vi "QuP Multiplexer Control.vi"() -> ()   [LabVIEW 2020, in "QuPMXdriver.lvlib"]
uses:
  QuPMXdriver.lvlib
  91754cce-ab52-4237-b78a-64c01c446f44.vi
  32ad12f4-2c8c-4504-800a-0d774754ae80.vi
  bf4f7028-8ca7-4759-aadb-7144e2be3c91.vi
  040f1b57-66c1-4072-aa26-6ea72dd8171f.vi
  6aed5eb3-691d-4dc6-b830-00691c629857.vi
  3345cd23-f609-4396-914e-6427162a2d46.vi
  Sequence Editor.vi
  <vilib>/Comparison/Equal/Equal Functor/Equal Functor.lvclass
panel:
  in  "Init-reset":bool caption="Reset after connect:"
  in  "Init-idquery":bool=TRUE caption="ID query after connect:"
  out "FPdisAcon":refnum<vi>[](array[refnum])
  in  "Startup delay (ms)":u32=2000
  in  "disconnect":bool
  out "dummy for event \"check channels\"":bool
  in  "Set to sequence line:":i32=2 min=1 step=1
  in  "set sq line":bool
  out "Connected\nboards":bool[](array[boolean])
  in  "Get sq from MX":bool
  in  "Load sq to MX":bool
  in  "no sequences get":bool
  out "Number of sequence lines:":i32 min=0 step=1
  in  "sequence editor":bool
  out "Guards ref array":refnum<vi>[][](array[refnum])
  in  "G5C1":bool
  in  "G5C2":bool
  in  "G6C1":bool
  in  "G6C2":bool
  in  "G4C1":bool
  in  "G4C2":bool
  in  "G3C1":bool
  in  "G3C2":bool
  in  "G2C1":bool
  in  "G2C2":bool
  in  "G1C1":bool
  in  "G1C2":bool
  out "No. of connected slave boards:":u32
  out "Slaves ref array":refnum<vi>[][](array[refnum])
  in  "S5C1":bool
  in  "S5C2":bool
  in  "S6C1":bool
  in  "S6C2":bool
  in  "S4C1":bool
  in  "S4C2":bool
  in  "S3C1":bool
  in  "S3C2":bool
  in  "S2C1":bool
  in  "S2C2":bool
  in  "S1C1":bool
  in  "S1C2":bool
  in  "connect":bool
  in  "Get Status":bool
  out "Ready?":bool=TRUE
  out "Enabled":bool=TRUE
  in  "check channels":bool
  in  "delay get":bool
  in  "delay set":bool
  in  "Enable\nDelay (ms)":dbl=2.0 min=0.8
  in  "timer get":bool
  in  "timer set":bool
  in  "Timer (ms)":i32=1000 min=0 step=1
  in  "Trigger polarity":enum32{"Positive", "Negative"}(radio)
  in  "Trigger source":enum32{"Internal", "External"}(radio)
  out "FPenAcon":refnum<vi>[](array[refnum])
  in  "Operation":enum32{"Remote", "Local"}(radio)=enum."Local"
  out "ID:":string
  in  "reset":bool
  in  "clear":bool
  in  "stop":bool
  in  "start":bool
  in  "resume":bool
  in  "pause":bool
  in  "Close":bool
  out "error":errorcluster
  in  "VISA":refnum<visa-resource-name>
  # "Connect"
  # "Status"
  # "Channels"
  # "Properties"
  # "Slave boards"
  # "1       2      3      4      5      6"
  # "Channel 1"
  # "Channel 2"
  # "1       2      3      4      5      6"
  # "Guards"
  # "Channel 1"
  # "These are buttons,\nclick it!"
  # "Channel 2"
  # "Sequence"
  # "Error"
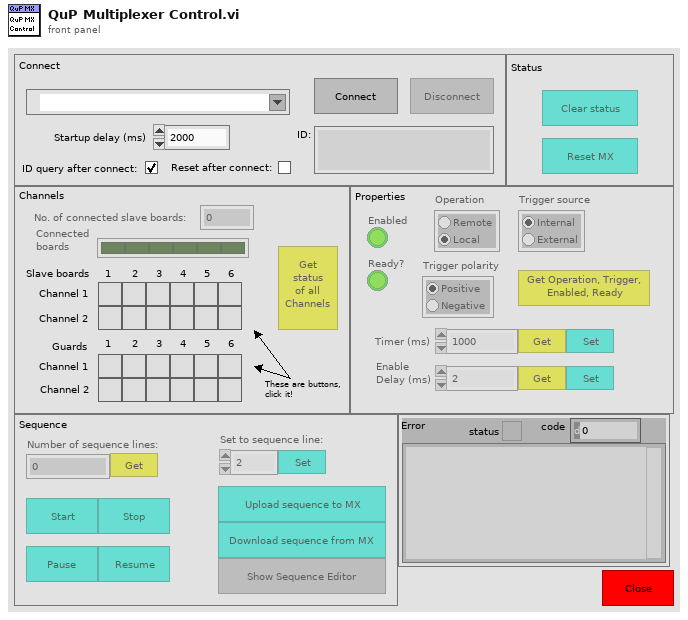
[diagram p1: front panel]
types:
  T1 = enum8{"Enabled", "Disabled", "Disabled and Grayed Out"}
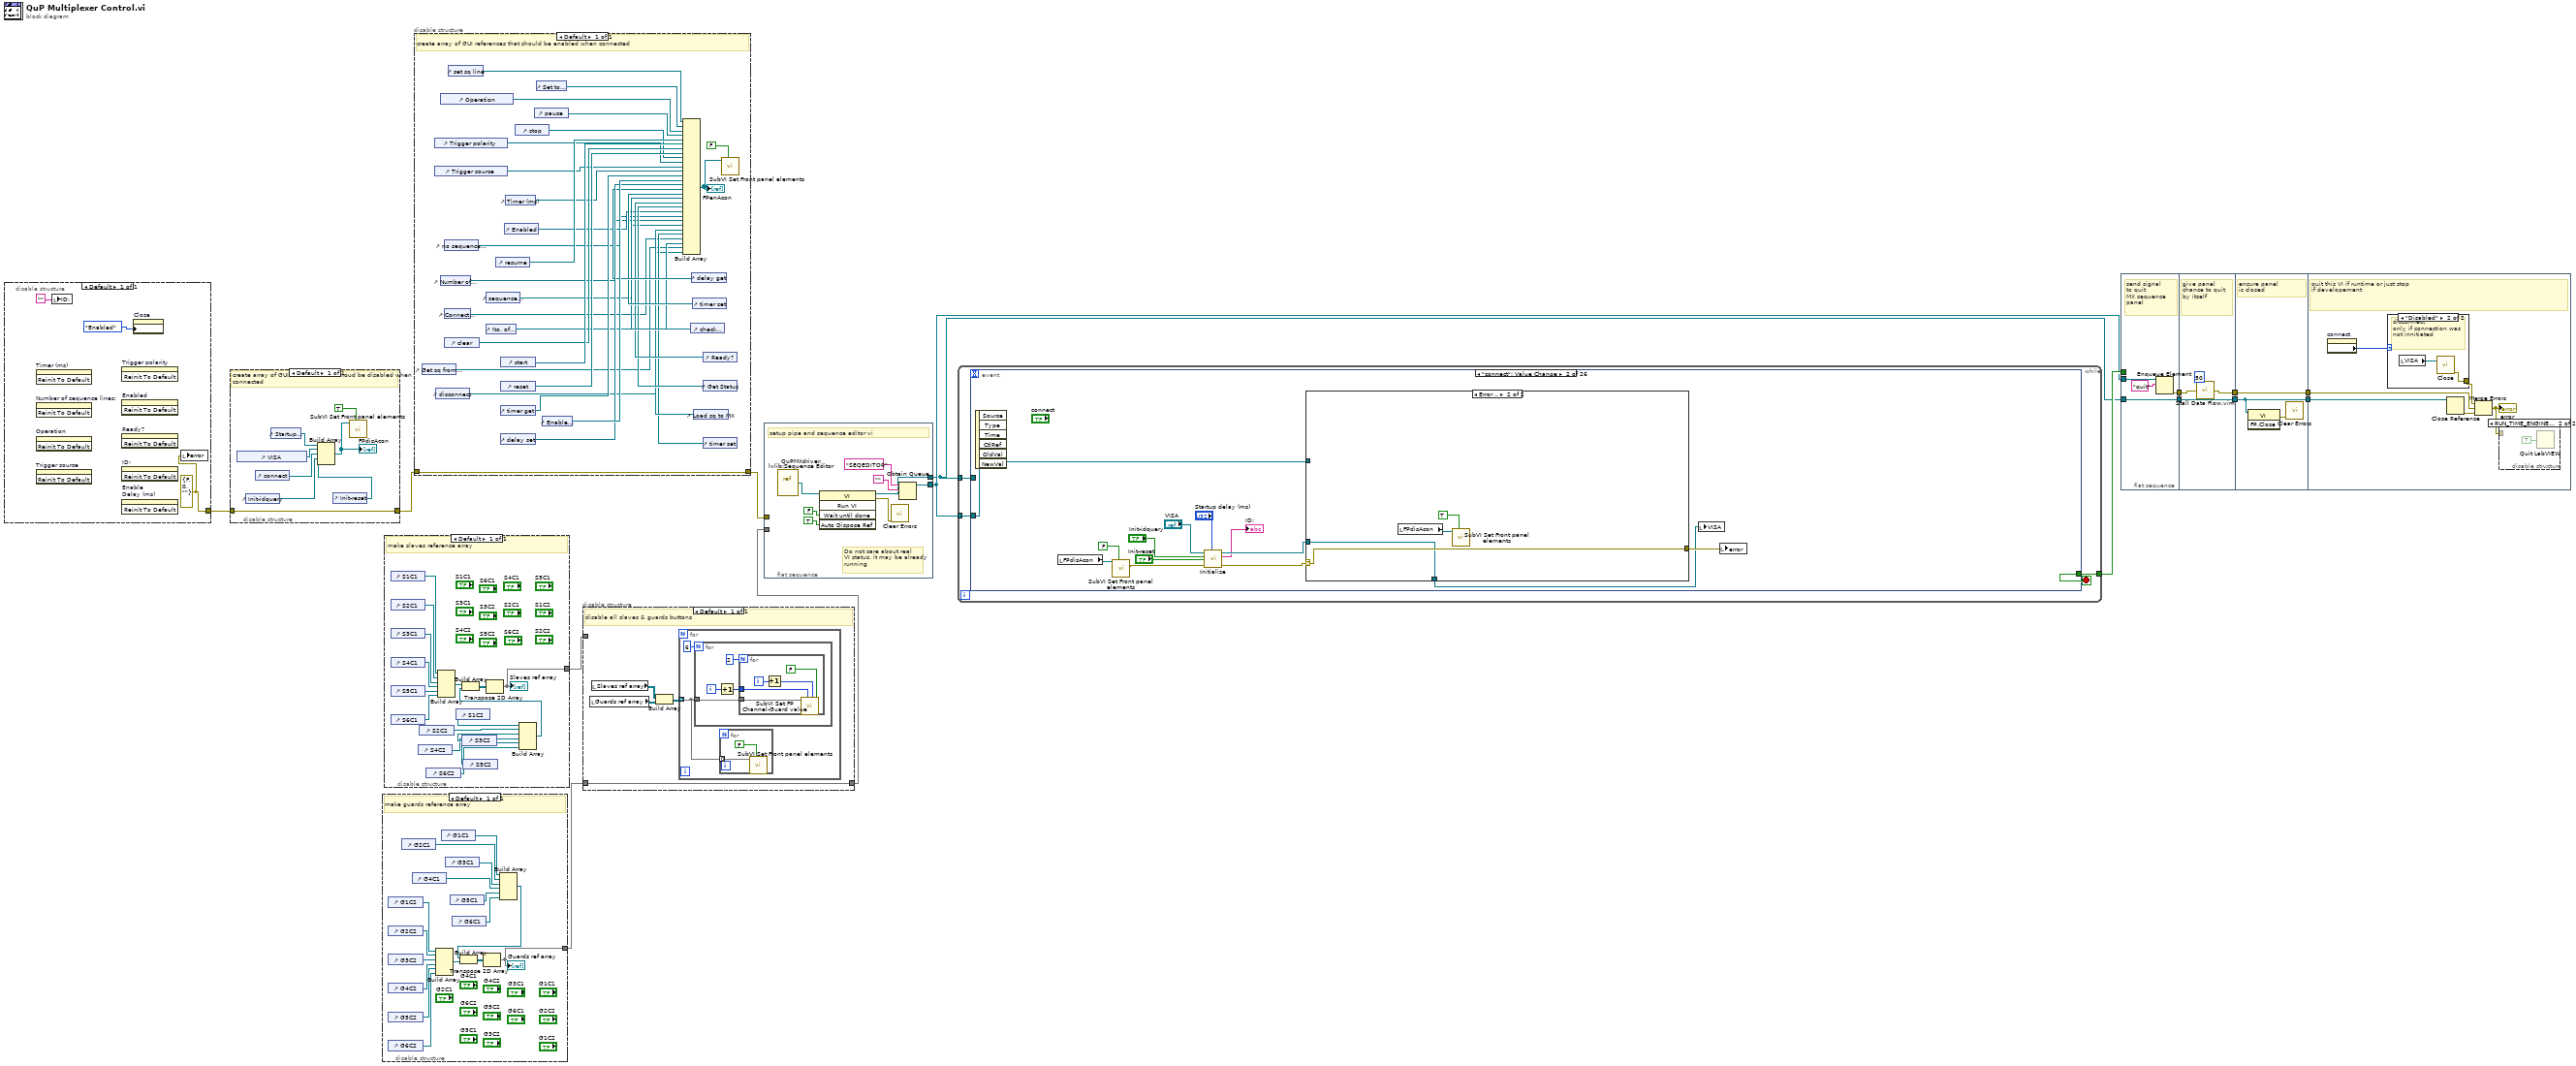
[diagram p0: block diagram]
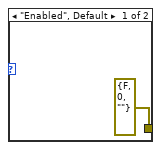
[diagram p2: hidden frame]
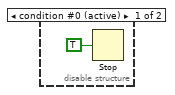
[diagram p3: hidden frame]
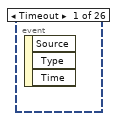
[diagram p4: hidden frame]
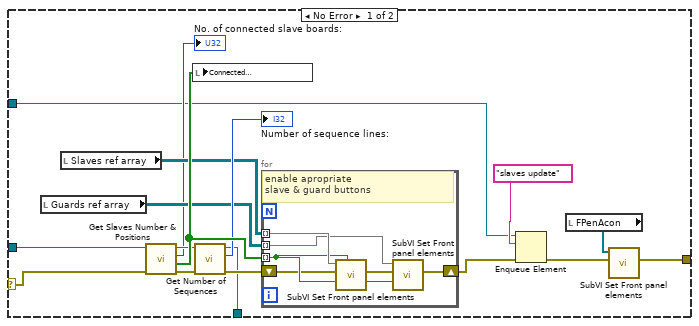
[diagram p5: hidden frame]
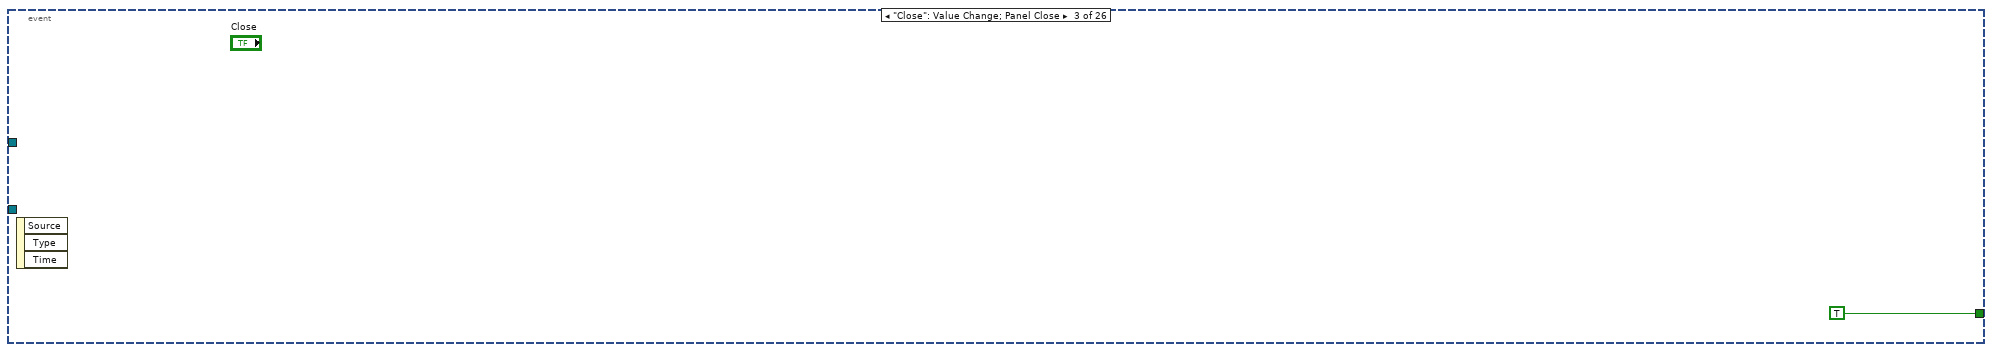
[diagram p6: hidden frame]
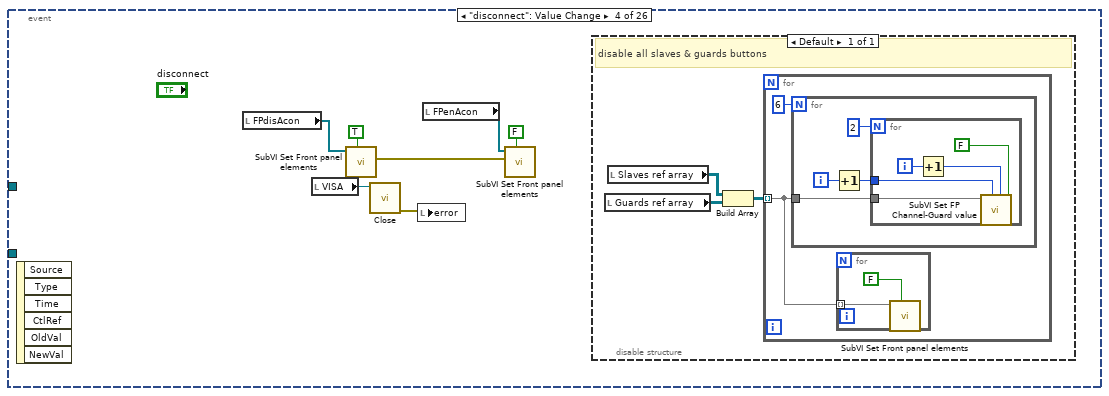
[diagram p7: hidden frame]
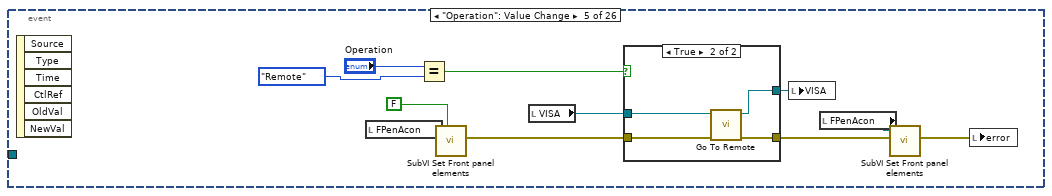
[diagram p8: hidden frame]
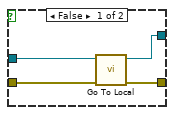
[diagram p9: hidden frame]
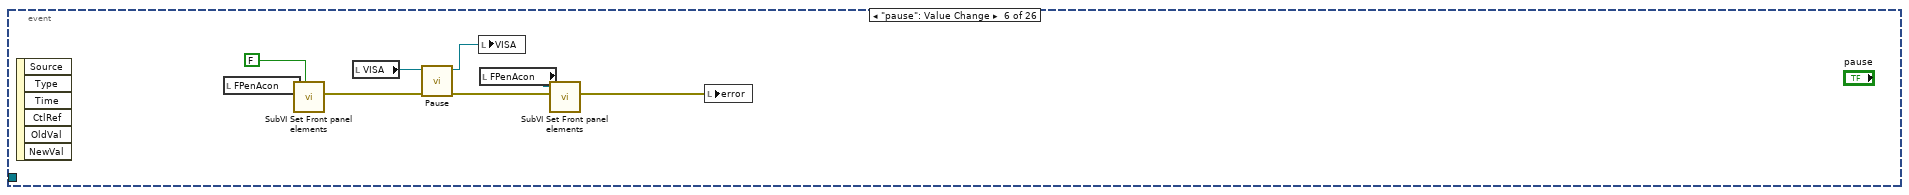
[diagram p10: hidden frame]
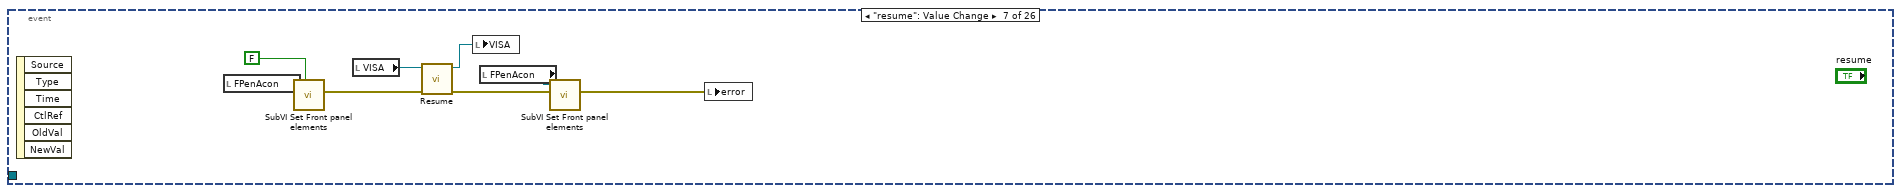
[diagram p11: hidden frame]
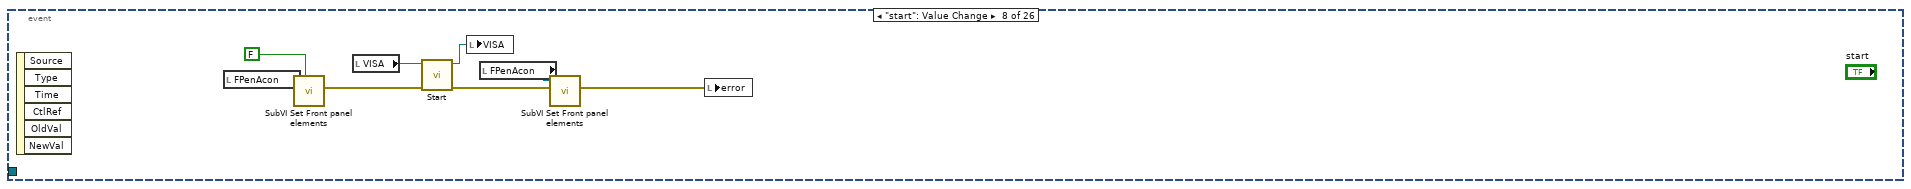
[diagram p12: hidden frame]
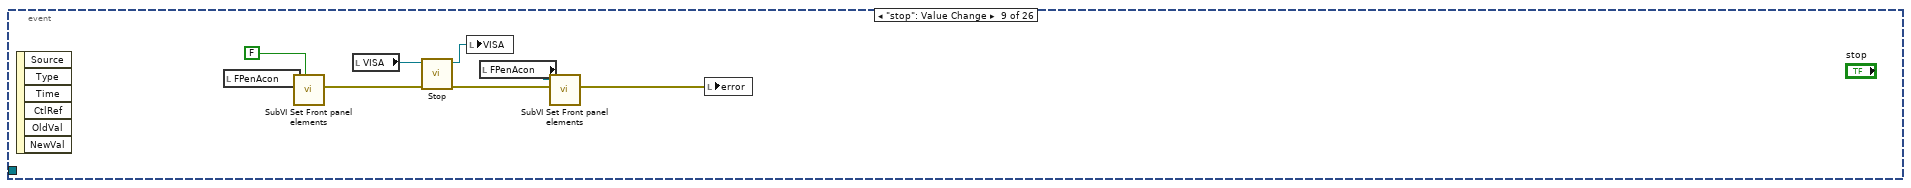
[diagram p13: hidden frame]
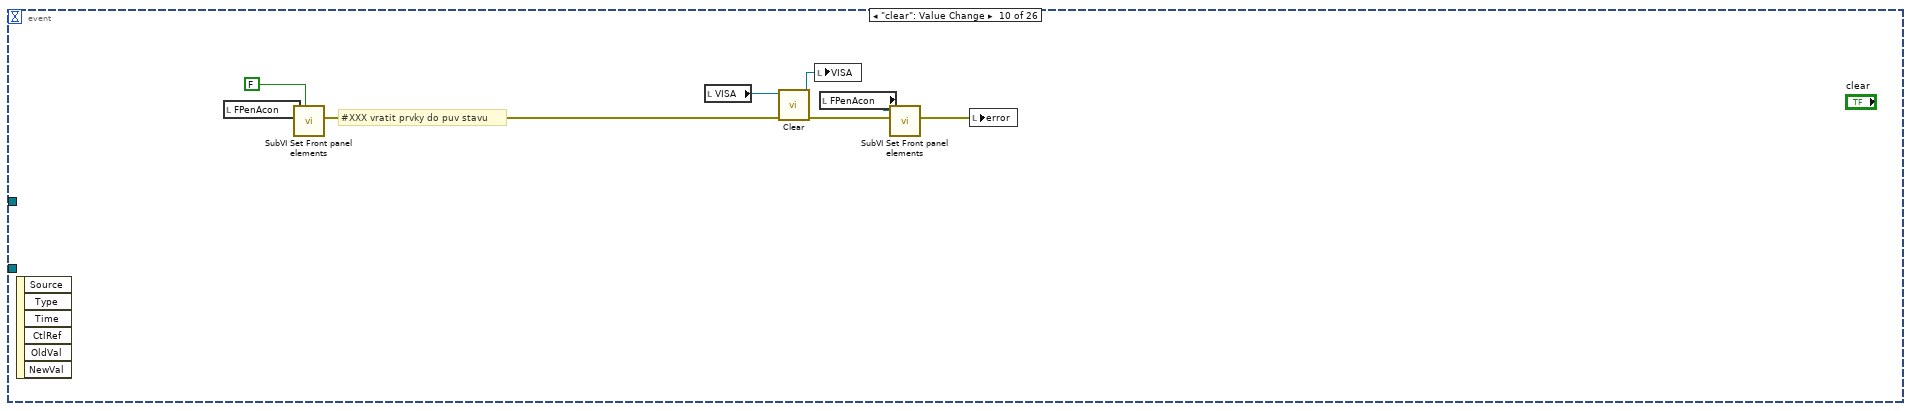
[diagram p14: hidden frame]
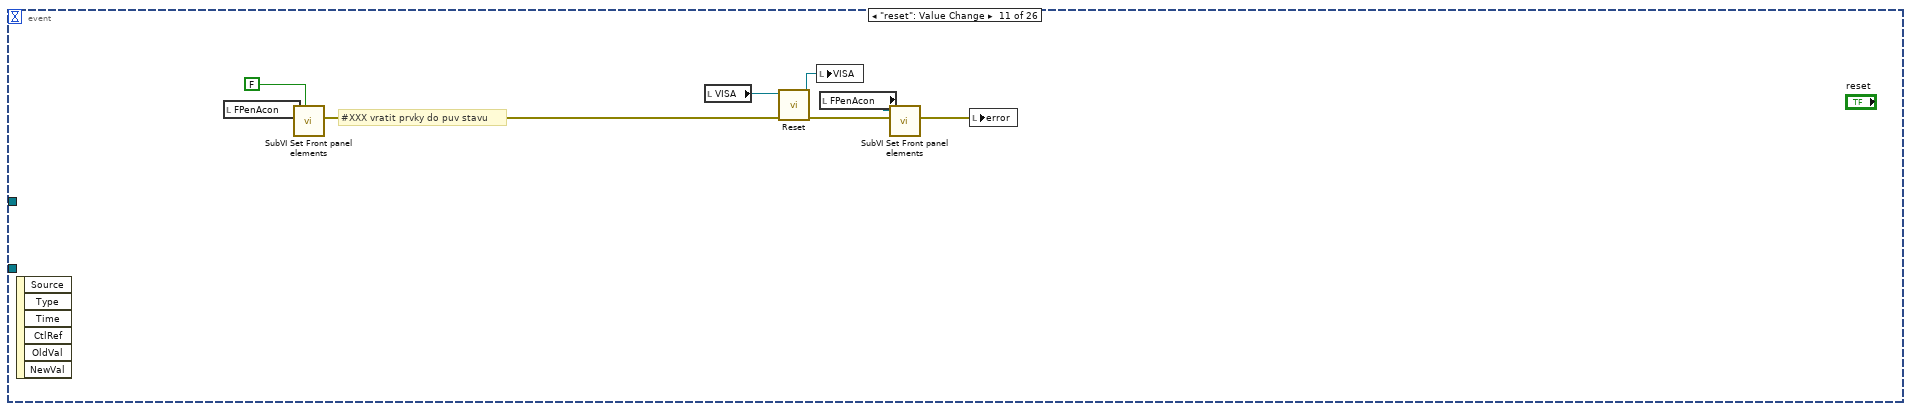
[diagram p15: hidden frame]
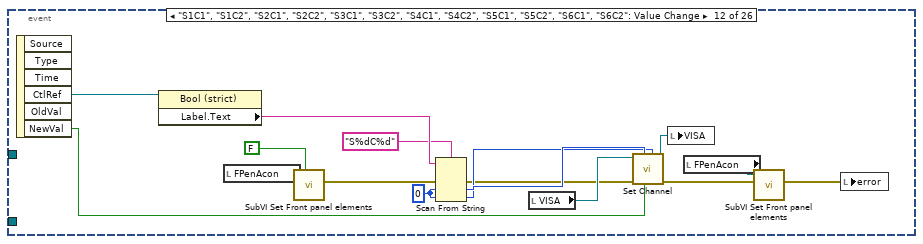
[diagram p16: hidden frame]
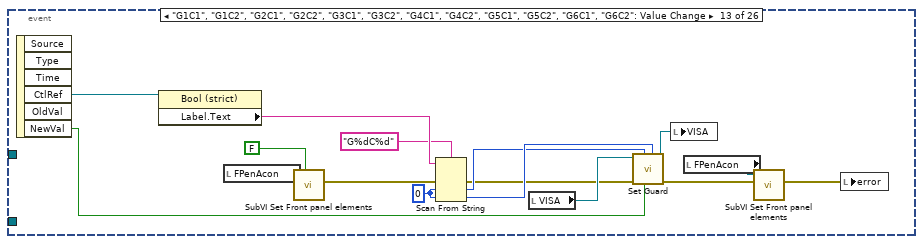
[diagram p17: hidden frame]
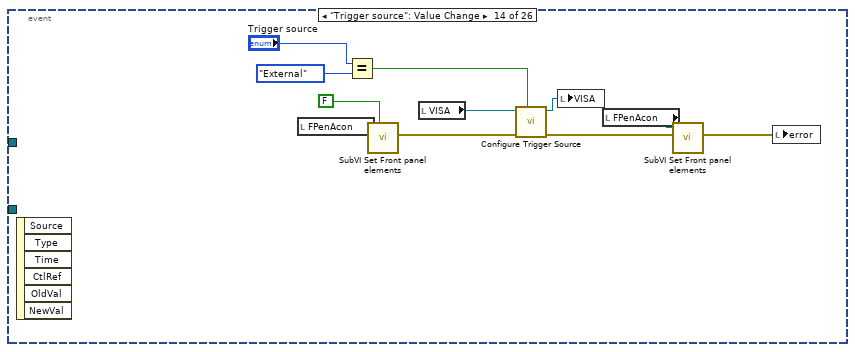
[diagram p18: hidden frame]
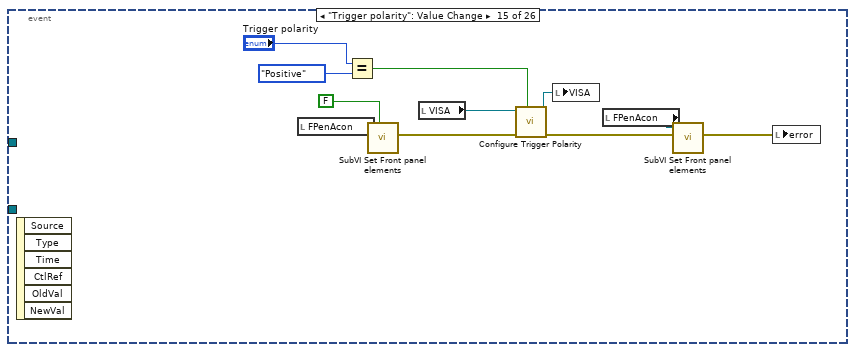
[diagram p19: hidden frame]
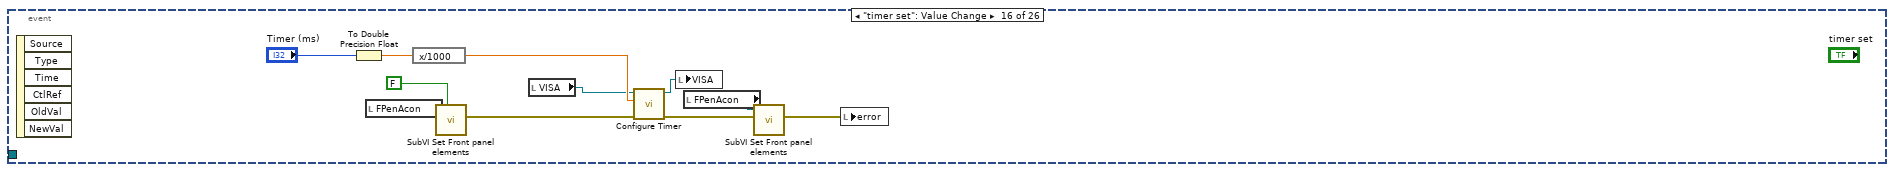
[diagram p20: hidden frame]
diagram:
  n1 = disable-structure shown="Default" {
    disable-tunnel: [w16] -> w5
    frame Enabled {
      w16 = errorcluster {"status"=FALSE, "code"=0, "source"=""} ("error in (no error)")
      n2 = invoke on="Timer (ms)" class="DigNum (strict)" method="Reinit To Default"() -> ()  [unwired: 3 in, 3 out]
      n3 = invoke on="Number of sequence lines:" class="DigNum (strict)" method="Reinit To Default"() -> ()  [unwired: 3 in, 3 out]
      n4 = invoke on="Operation" class="RadioBtnsControl (strict)" method="Reinit To Default"() -> ()  [unwired: 3 in, 3 out]
      n5 = invoke on="Trigger source" class="RadioBtnsControl (strict)" method="Reinit To Default"() -> ()  [unwired: 3 in, 3 out]
      n6 = local write "ID:"("") -> ()
      n7 = invoke on="Trigger polarity" class="RadioBtnsControl (strict)" method="Reinit To Default"() -> ()  [unwired: 3 in, 3 out]
      n8 = invoke on="Enabled" class="Bool (strict)" method="Reinit To Default"() -> ()  [unwired: 3 in, 3 out]
      n9 = invoke on="Ready?" class="Bool (strict)" method="Reinit To Default"() -> ()  [unwired: 3 in, 3 out]
      n10 = invoke on="ID:" class="Str" method="Reinit To Default"() -> ()  [unwired: 3 in, 3 out]
      n11 = invoke on="Enable\nDelay (ms)" class="DigNum (strict)" method="Reinit To Default"() -> ()  [unwired: 3 in, 3 out]
      n12 = property on="Close" class="Bool"("DisabledEnum"=T1."Enabled" ("Disabled")) -> ()  [unwired: 2 in, 2 out]
      n13 = local write "error"(w16) -> ()
    }
  }
  n14 = disable-structure shown="Default" {
    disable-tunnel: [w21] -> w6
    disable-tunnel: w5 -> [w21]
    frame Enabled {
      # "create array of GUI references that shoud be disabled when connected"
      n15 = control-ref of="VISA"() -> (w25:refnum<vi>)
      n16 = control-ref of="Init-idquery"() -> (w20:refnum<vi>)
      n17 = control-ref of="connect"() -> (w24:refnum<vi>)
      n18 = control-ref of="Startup delay (ms)"() -> (w26:refnum<vi>)
      n19 = control-ref of="Init-reset"() -> (w19:refnum<vi>)
      n20 = Build Array(w26, w25, w24, w20, w19) -> (w22:refnum<vi>[])
      "FPdisAcon" <- w22
      n21 = call "SubVI Set Front panel elements.vi"("Enable elements (T)"=TRUE ("Enable elements"), "Array"=w22) -> ()  [unwired: 9 in, 1 out]
    }
  }
  n22 = disable-structure shown="Default" {
    disable-tunnel: [w27] -> w13
    frame Enabled {
      # "make guards reference array"
      n23 = control-ref of="G1C2"() -> (w28:refnum<vi>)
      n24 = control-ref of="G2C2"() -> (w29:refnum<vi>)
      n25 = control-ref of="G3C2"() -> (w30:refnum<vi>)
      n26 = control-ref of="G4C2"() -> (w31:refnum<vi>)
      n27 = control-ref of="G5C2"() -> (w32:refnum<vi>)
      n28 = control-ref of="G6C2"() -> (w33:refnum<vi>)
      n29 = control-ref of="G2C1"() -> (w36:refnum<vi>)
      n30 = control-ref of="G4C1"() -> (w38:refnum<vi>)
      n31 = Build Array(w28, w29, w30, w31, w32, w33) -> (w41:refnum<vi>[])
      n32 = control-ref of="G1C1"() -> (w35:refnum<vi>)
      n33 = control-ref of="G3C1"() -> (w37:refnum<vi>)
      n34 = control-ref of="G5C1"() -> (w39:refnum<vi>)
      n35 = control-ref of="G6C1"() -> (w40:refnum<vi>)
      n36 = Build Array(w35, w36, w37, w38, w39, w40) -> (w34:refnum<vi>[])
      n37 = Build Array(w34, w41) -> (w42:refnum<vi>[][])
      n38 = Transpose 2D Array(2D array=w42) -> (transposed array=w27:refnum<vi>[][])
      "Guards ref array" <- w27
    }
  }
  n39 = disable-structure shown="Default" {
    disable-tunnel: [w43] -> w14
    frame Enabled {
      # "make slaves reference array"
      n40 = control-ref of="S1C1"() -> (w58:refnum<vi>)
      n41 = control-ref of="S2C1"() -> (w57:refnum<vi>)
      n42 = control-ref of="S3C1"() -> (w56:refnum<vi>)
      n43 = control-ref of="S4C1"() -> (w55:refnum<vi>)
      n44 = control-ref of="S5C1"() -> (w54:refnum<vi>)
      n45 = control-ref of="S6C1"() -> (w53:refnum<vi>)
      n46 = control-ref of="S4C2"() -> (w49:refnum<vi>)
      n47 = control-ref of="S2C2"() -> (w51:refnum<vi>)
      n48 = control-ref of="S6C2"() -> (w47:refnum<vi>)
      n49 = Build Array(w58, w57, w56, w55, w54, w53) -> (w45:refnum<vi>[])
      n50 = control-ref of="S1C2"() -> (w52:refnum<vi>)
      n51 = control-ref of="S3C2"() -> (w50:refnum<vi>)
      n52 = control-ref of="S5C2"() -> (w48:refnum<vi>)
      n53 = Build Array(w52, w51, w50, w49, w48, w47) -> (w46:refnum<vi>[])
      n54 = Build Array(w45, w46) -> (w44:refnum<vi>[][])
      n55 = Transpose 2D Array(2D array=w44) -> (transposed array=w43:refnum<vi>[][])
      "Slaves ref array" <- w43
    }
  }
  n56 = disable-structure shown="Default" {
    disable-tunnel: [w66] -> w9
    disable-tunnel: w6 -> [w66]
    frame Enabled {
      # "create array of GUI references that should be enabled when connected"
      n57 = control-ref of="Get sq from MX"() -> (w62:refnum<vi>)
      n58 = control-ref of="Trigger polarity"() -> (w82:refnum<vi>)
      n59 = control-ref of="Trigger source"() -> (w81:refnum<vi>)
      n60 = control-ref of="disconnect"() -> (w59:refnum<vi>)
      n61 = control-ref of="Operation"() -> (w91:refnum<vi>)
      n62 = control-ref of="Number of sequence lines:"() -> (w69:refnum<vi>)
      n63 = control-ref of="no sequences get"() -> (w70:refnum<vi>)
      n64 = control-ref of="Connected\nboards"() -> (w64:refnum<vi>)
      n65 = control-ref of="clear"() -> (w87:refnum<vi>)
      n66 = control-ref of="set sq line"() -> (w60:refnum<vi>)
      n67 = control-ref of="sequence editor"() -> (w68:refnum<vi>)
      n68 = control-ref of="No. of connected slave boards:"() -> (w63:refnum<vi>)
      n69 = control-ref of="resume"() -> (w89:refnum<vi>)
      n70 = control-ref of="start"() -> (w88:refnum<vi>)
      n71 = control-ref of="reset"() -> (w86:refnum<vi>)
      n72 = control-ref of="timer get"() -> (w79:refnum<vi>)
      n73 = control-ref of="delay set"() -> (w77:refnum<vi>)
      n74 = control-ref of="Enabled"() -> (w71:refnum<vi>)
      n75 = control-ref of="Timer (ms)"() -> (w80:refnum<vi>)
      n76 = control-ref of="stop"() -> (w83:refnum<vi>)
      n77 = control-ref of="pause"() -> (w90:refnum<vi>)
      n78 = control-ref of="Set to sequence line:"() -> (w61:refnum<vi>)
      n79 = control-ref of="Enable\nDelay (ms)"() -> (w78:refnum<vi>)
      n80 = control-ref of="check channels"() -> (w74:refnum<vi>)
      n81 = control-ref of="delay get"() -> (w76:refnum<vi>)
      n82 = control-ref of="timer set"() -> (w75:refnum<vi>)
      n83 = control-ref of="Load sq to MX"() -> (w67:refnum<vi>)
      n84 = control-ref of="Ready?"() -> (w73:refnum<vi>)
      n85 = control-ref of="Get Status"() -> (w72:refnum<vi>)
      n86 = control-ref of="timer set"() -> (w65:refnum<vi>)
      n87 = Build Array(w60, w61, w91, w90, w89, w88, w87, w86, w83, w82, w81, w80, w79, w78, w77, w76, w75, w74, w73, w72, w71, w70, w69, w68, w67, w65, w64, w63, w62, w59) -> (w85:refnum<vi>[])
      "FPenAcon" <- w85
      n88 = call "SubVI Set Front panel elements.vi"("Enable elements (T)"=FALSE ("Enable elements"), "Array"=w85) -> ()  [unwired: 9 in, 1 out]
    }
  }
  n89 = disable-structure shown="Default" {
    disable-tunnel: w14 -> [_]
    disable-tunnel: w13 -> [w92]
    disable-tunnel: [w92] -> w10
    frame Enabled {
      # "disable all slaves & guards buttons"
      n90 = local read "Guards ref array"() -> (w93:refnum<vi>[][])
      n91 = local read "Slaves ref array"() -> (w95:refnum<vi>[][])
      n92 = Build Array(w95, w93) -> (w94:refnum<vi>[][][])
      n93 = for {
        tunnel: w94 -> [w96] mode=indexing
        n94 = for {
          N: 6 -> [_]
          tunnel: w96 -> [w101]
          i -> [w99]
          n95 = Increment(x=w99) -> (x+1=w98:i32)
          n96 = for {
            N: 2 -> [_]
            tunnel: w101 -> [w106]
            tunnel: w98 -> [w104]
            i -> [w103]
            n97 = Increment(x=w103) -> (x+1=w102:i32)
            n98 = call "SubVI Set FP Channel-Guard value.vi"("Value"=FALSE, "Ch ID"=w102, "Slave ID"=w104, "Slaves ref array"=w106) -> ()  [unwired: 7 in, 1 out]
          }
        }
        n99 = for {
          tunnel: w96 -> [w108] mode=indexing
          n100 = call "SubVI Set Front panel elements.vi"("Enable elements (T)"=FALSE, "Array"=w108) -> ()  [unwired: 9 in, 1 out]
        }
      }
    }
  }
  n101 = flat-sequence {
    tunnel: [w110] -> w12
    tunnel: [w112] -> w11
    tunnel: w10 -> [_]
    tunnel: w9 -> [_]
    frame #0 {
      # "Do not care about real\nVI status, it may be already\nrunning"
      # "setup pipe and sequence editor vi"
      n102 = vi-ref "QuPMXdriver.lvlib:Sequence Editor.vi"() -> (w116:refnum<vi>)
      n103 = invoke class="VI" method="Run VI"(reference=w116, "Wait until done"=FALSE ("Wait Until Done"), "Auto Dispose Ref"=TRUE ("Wait Until Done")) -> (reference out=w112:refnum<vi>, error out=w109:errorcluster)  [unwired: 2 in, 3 out]
      n104 = call <vilib>:"Clear Errors.vi"("error in (no error)"=w109) -> ()  [unwired: 5 in, 2 out]
      n105 = Obtain Queue(name (unnamed)="SEQEDITOR", element data type="") -> (queue out=w110:refnum<queue>)  [unwired: 3 in, 2 out]
    }
  }
  n106 = while {
    tunnel: [w119] -> w15
    tunnel: w12 -> [w118]
    tunnel: w11 -> [w117]
    stop <- w119 stop-if-true
    n107 = event shown="[1] \"connect\": Value Change" {
      selector: _ -> [_ _ _ _ _ _ _ _ _ _ _ _ _ _ _ _ _ _ _ _ _ _ _ _ _ _]
      dyn-events: _ -> [_ _ _ _ _ _ _ _ _ _ _ _ _ _ _ _ _ _ _ _ _ _ _ _ _ _]
      timeout: _ -> [_ _ _ _ _ _ _ _ _ _ _ _ _ _ _ _ _ _ _ _ _ _ _ _ _ _]
      tunnel: [_ _ TRUE ("Stop") _ _ _ _ _ _ _ _ _ _ _ _ _ _ _ _ _ _ _ _ _ _ _] -> w119
      tunnel: w118 -> [_ w129 _ _ _ _ _ _ _ _ _ _ _ _ _ _ _ _ _ w350 _ _ w419 _ _ w499]
      tunnel: w117 -> [_ _ _ _ _ _ _ _ _ _ _ _ _ _ _ _ _ _ _ _ _ _ _ w424 w474 w502]
      event Timeout {
        n108 = event-data() -> ()  [unwired: 1 in, 3 out]
      }
      event "connect": Value Change {
        n109 = event-data() -> ()  [unwired: 1 in, 6 out]
        n110 = local read "FPdisAcon"() -> (w126:refnum<vi>[])
        n111 = call "SubVI Set Front panel elements.vi"("Enable elements (T)"=FALSE, "Array"=w126) -> ("error out"=w124:errorcluster)  [unwired: 9 in]
        n112 = call "Initialize.vi"("Startup delay (0 ms)"="Startup delay (ms)", "error in (no error)"=w124, "Reset (False)"="Init-reset", "ID Query (True)"="Init-idquery", "VISA resource name"="VISA") -> ("error out"=w123:errorcluster, "ID"=→"ID:":string, "VISA resource name out"=w131:refnum<visa-resource-name>)  [unwired: 4 in]
        n113 = case shown="Error .." w123 {
          selector: w123 -> [w134 w159]
          tunnel: w131 -> [w141 w156]
          tunnel: w129 -> [w136 _]
          tunnel: [w135 w159] -> w127
          tunnel: [w133 w156] -> w120
          frame No Error {
            n114 = local read "Guards ref array"() -> (w144:refnum<vi>[][])
            n115 = local read "Slaves ref array"() -> (w143:refnum<vi>[][])
            n116 = call "Get Slaves Number & Positions.vi"("error in (no error)"=w134, "VISA resource name"=w141) -> ("error out"=w145:errorcluster, "Connected Slaves"=w149:bool[], "No. of Slaves"=→"No. of connected slave boards:":u32, "VISA resource name out"=w147:refnum<visa-resource-name>)  [unwired: 6 in]
            n117 = local write "Connected\nboards"(w149) -> ()
            n118 = call "Get Number of Sequences.vi"("error in (no error)"=w145, "VISA resource name"=w147) -> ("error out"=w146:errorcluster, "Number of sequences"=→"Number of sequence lines:":i32, "VISA resource name out"=w133:refnum<visa-resource-name>)  [unwired: 7 in]
            n119 = for {
              tunnel: w143 -> [w155] mode=indexing
              tunnel: w149 -> [w153] mode=indexing
              tunnel: w144 -> [w154] mode=indexing
              shift-right: [w151] -> w137
              shift-left: w146 -> [w150]
              # "enable apropriate\nslave & guard buttons"
              n120 = call "SubVI Set Front panel elements.vi"("Enable elements (T)"=w153, "error in (passthrough)"=w150, "Array"=w155) -> ("error out"=w152:errorcluster)  [unwired: 8 in]
              n121 = call "SubVI Set Front panel elements.vi"("Enable elements (T)"=w153, "error in (passthrough)"=w152, "Array"=w154) -> ("error out"=w151:errorcluster)  [unwired: 8 in]
            }
            n122 = Enqueue Element(queue=w136, element="slaves update", error in (no error)=w137) -> (error out=w140:errorcluster)  [unwired: 1 in, 2 out]
            n123 = local read "FPenAcon"() -> (w139:refnum<vi>[])
            n124 = call "SubVI Set Front panel elements.vi"("error in (passthrough)"=w140, "Array"=w139) -> ("error out"=w135:errorcluster)  [unwired: 9 in]
          }
          frame Error {
            n125 = local read "FPdisAcon"() -> (w157:refnum<vi>[])
            n126 = call "SubVI Set Front panel elements.vi"("Enable elements (T)"=TRUE, "Array"=w157) -> ()  [unwired: 9 in, 1 out]
          }
        }
        n127 = local write "VISA"(w120) -> ()
        n128 = local write "error"(w127) -> ()
      }
      event "Close": Value Change; Panel Close {
        n129 = event-data() -> ()  [unwired: 1 in, 3 out]
      }
      event "disconnect": Value Change {
        n130 = event-data() -> ()  [unwired: 1 in, 6 out]
        n131 = local read "FPdisAcon"() -> (w162:refnum<vi>[])
        n132 = local read "VISA"() -> (w167:refnum<visa-resource-name>)
        n133 = call "SubVI Set Front panel elements.vi"("Enable elements (T)"=TRUE, "Array"=w162) -> ("error out"=w163:errorcluster)  [unwired: 9 in]
        n134 = call "Close.vi"("VISA resource name"=w167) -> ("error out"=w166:errorcluster)  [unwired: 10 in]
        n135 = local write "error"(w166) -> ()
        n136 = local read "FPenAcon"() -> (w165:refnum<vi>[])
        n137 = call "SubVI Set Front panel elements.vi"("Enable elements (T)"=FALSE, "error in (passthrough)"=w163, "Array"=w165) -> ()  [unwired: 8 in, 1 out]
        n138 = disable-structure shown="Default" {
          frame Enabled {
            # "disable all slaves & guards buttons"
            n139 = local read "Guards ref array"() -> (w168:refnum<vi>[][])
            n140 = local read "Slaves ref array"() -> (w170:refnum<vi>[][])
            n141 = Build Array(w170, w168) -> (w169:refnum<vi>[][][])
            n142 = for {
              tunnel: w169 -> [w171] mode=indexing
              n143 = for {
                N: 6 -> [_]
                tunnel: w171 -> [w176]
                i -> [w174]
                n144 = Increment(x=w174) -> (x+1=w173:i32)
                n145 = for {
                  N: 2 -> [_]
                  tunnel: w176 -> [w181]
                  tunnel: w173 -> [w179]
                  i -> [w178]
                  n146 = Increment(x=w178) -> (x+1=w177:i32)
                  n147 = call "SubVI Set FP Channel-Guard value.vi"("Value"=FALSE, "Ch ID"=w177, "Slave ID"=w179, "Slaves ref array"=w181) -> ()  [unwired: 7 in, 1 out]
                }
              }
              n148 = for {
                tunnel: w171 -> [w183] mode=indexing
                n149 = call "SubVI Set Front panel elements.vi"("Enable elements (T)"=FALSE, "Array"=w183) -> ()  [unwired: 9 in, 1 out]
              }
            }
          }
        }
      }
      event "Operation": Value Change {
        n150 = event-data() -> ()  [unwired: 1 in, 6 out]
        n151 = local read "FPenAcon"() -> (w190:refnum<vi>[])
        n152 = Equal?(x="Operation", y=enum32{"Remote", "Local"}."Remote") -> (x = y?=w191:bool)
        n153 = call "SubVI Set Front panel elements.vi"("Enable elements (T)"=FALSE, "Array"=w190) -> ("error out"=w188:errorcluster)  [unwired: 9 in]
        n154 = local read "VISA"() -> (w194:refnum<visa-resource-name>)
        n155 = case shown="True" w191 {
          tunnel: [w198 w202] -> w187
          tunnel: w194 -> [w197 w201]
          tunnel: w188 -> [w196 w200]
          tunnel: [w195 w199] -> w184
          frame False {
            n156 = call "Go To Local.vi"("error in (no error)"=w196, "VISA resource name"=w197) -> ("error out"=w198:errorcluster, "VISA resource name out"=w195:refnum<visa-resource-name>)  [unwired: 8 in]
          }
          frame True {
            n157 = call "Go To Remote.vi"("error in (no error)"=w200, "VISA resource name"=w201) -> ("error out"=w202:errorcluster, "VISA resource name out"=w199:refnum<visa-resource-name>)  [unwired: 8 in]
          }
        }
        n158 = local write "VISA"(w184) -> ()
        n159 = local read "FPenAcon"() -> (w185:refnum<vi>[])
        n160 = call "SubVI Set Front panel elements.vi"("error in (passthrough)"=w187, "Array"=w185) -> ("error out"=w186:errorcluster)  [unwired: 9 in]
        n161 = local write "error"(w186) -> ()
      }
      event "pause": Value Change {
        n162 = event-data() -> ()  [unwired: 1 in, 6 out]
        n163 = local read "FPenAcon"() -> (w209:refnum<vi>[])
        n164 = call "SubVI Set Front panel elements.vi"("Enable elements (T)"=FALSE, "Array"=w209) -> ("error out"=w206:errorcluster)  [unwired: 9 in]
        n165 = local read "VISA"() -> (w210:refnum<visa-resource-name>)
        n166 = call "Pause.vi"("error in (no error)"=w206, "VISA resource name"=w210) -> ("error out"=w205:errorcluster, "VISA resource name out"=w203:refnum<visa-resource-name>)  [unwired: 8 in]
        n167 = local write "VISA"(w203) -> ()
        n168 = local read "FPenAcon"() -> (w207:refnum<vi>[])
        n169 = call "SubVI Set Front panel elements.vi"("error in (passthrough)"=w205, "Array"=w207) -> ("error out"=w204:errorcluster)  [unwired: 9 in]
        n170 = local write "error"(w204) -> ()
      }
      event "resume": Value Change {
        n171 = event-data() -> ()  [unwired: 1 in, 6 out]
        n172 = local read "FPenAcon"() -> (w216:refnum<vi>[])
        n173 = call "SubVI Set Front panel elements.vi"("Enable elements (T)"=FALSE, "Array"=w216) -> ("error out"=w214:errorcluster)  [unwired: 9 in]
        n174 = local read "VISA"() -> (w218:refnum<visa-resource-name>)
        n175 = call "Resume.vi"("error in (no error)"=w214, "VISA resource name"=w218) -> ("error out"=w213:errorcluster, "VISA resource name out"=w211:refnum<visa-resource-name>)  [unwired: 8 in]
        n176 = local write "VISA"(w211) -> ()
        n177 = local read "FPenAcon"() -> (w217:refnum<vi>[])
        n178 = call "SubVI Set Front panel elements.vi"("error in (passthrough)"=w213, "Array"=w217) -> ("error out"=w212:errorcluster)  [unwired: 9 in]
        n179 = local write "error"(w212) -> ()
      }
      event "start": Value Change {
        n180 = event-data() -> ()  [unwired: 1 in, 6 out]
        n181 = local read "FPenAcon"() -> (w224:refnum<vi>[])
        n182 = call "SubVI Set Front panel elements.vi"("Enable elements (T)"=FALSE, "Array"=w224) -> ("error out"=w222:errorcluster)  [unwired: 9 in]
        n183 = local read "VISA"() -> (w226:refnum<visa-resource-name>)
        n184 = call "Start.vi"("error in (no error)"=w222, "VISA resource name"=w226) -> ("error out"=w221:errorcluster, "VISA resource name out"=w219:refnum<visa-resource-name>)  [unwired: 8 in]
        n185 = local write "VISA"(w219) -> ()
        n186 = local read "FPenAcon"() -> (w225:refnum<vi>[])
        n187 = call "SubVI Set Front panel elements.vi"("error in (passthrough)"=w221, "Array"=w225) -> ("error out"=w220:errorcluster)  [unwired: 9 in]
        n188 = local write "error"(w220) -> ()
      }
      event "stop": Value Change {
        n189 = event-data() -> ()  [unwired: 1 in, 6 out]
        n190 = local read "FPenAcon"() -> (w232:refnum<vi>[])
        n191 = call "SubVI Set Front panel elements.vi"("Enable elements (T)"=FALSE, "Array"=w232) -> ("error out"=w230:errorcluster)  [unwired: 9 in]
        n192 = local read "VISA"() -> (w234:refnum<visa-resource-name>)
        n193 = call "Stop.vi"("error in (no error)"=w230, "VISA resource name"=w234) -> ("error out"=w229:errorcluster, "VISA resource name out"=w227:refnum<visa-resource-name>)  [unwired: 8 in]
        n194 = local write "VISA"(w227) -> ()
        n195 = local read "FPenAcon"() -> (w233:refnum<vi>[])
        n196 = call "SubVI Set Front panel elements.vi"("error in (passthrough)"=w229, "Array"=w233) -> ("error out"=w228:errorcluster)  [unwired: 9 in]
        n197 = local write "error"(w228) -> ()
      }
      event "clear": Value Change {
        # "#XXX vratit prvky do puv stavu"
        n198 = event-data() -> ()  [unwired: 1 in, 6 out]
        n199 = local read "FPenAcon"() -> (w240:refnum<vi>[])
        n200 = call "SubVI Set Front panel elements.vi"("Enable elements (T)"=FALSE, "Array"=w240) -> ("error out"=w238:errorcluster)  [unwired: 9 in]
        n201 = local read "VISA"() -> (w242:refnum<visa-resource-name>)
        n202 = call "Clear.vi"("error in (no error)"=w238, "VISA resource name"=w242) -> ("error out"=w237:errorcluster, "VISA resource name out"=w235:refnum<visa-resource-name>)  [unwired: 8 in]
        n203 = local write "VISA"(w235) -> ()
        n204 = local read "FPenAcon"() -> (w241:refnum<vi>[])
        n205 = call "SubVI Set Front panel elements.vi"("error in (passthrough)"=w237, "Array"=w241) -> ("error out"=w236:errorcluster)  [unwired: 9 in]
        n206 = local write "error"(w236) -> ()
      }
      event "reset": Value Change {
        # "#XXX vratit prvky do puv stavu"
        n207 = event-data() -> ()  [unwired: 1 in, 6 out]
        n208 = local read "FPenAcon"() -> (w248:refnum<vi>[])
        n209 = call "SubVI Set Front panel elements.vi"("Enable elements (T)"=FALSE, "Array"=w248) -> ("error out"=w246:errorcluster)  [unwired: 9 in]
        n210 = local read "VISA"() -> (w250:refnum<visa-resource-name>)
        n211 = call "Reset.vi"("error in (no error)"=w246, "VISA resource name"=w250) -> ("error out"=w245:errorcluster, "VISA resource name out"=w243:refnum<visa-resource-name>)  [unwired: 8 in]
        n212 = local write "VISA"(w243) -> ()
        n213 = local read "FPenAcon"() -> (w249:refnum<vi>[])
        n214 = call "SubVI Set Front panel elements.vi"("error in (passthrough)"=w245, "Array"=w249) -> ("error out"=w244:errorcluster)  [unwired: 9 in]
        n215 = local write "error"(w244) -> ()
      }
      event "S1C1", "S1C2", "S2C1", "S2C2", "S3C1", "S3C2", "S4C1", "S4C2", "S5C1", "S5C2", "S6C1", "S6C2": Value Change {
        w252 = 0 ("default value 1")
        n216 = event-data() -> ("CtlRef"=w266:refnum<vi>, "NewVal"=w260:bool)  [unwired: 1 in, 4 out]
        n217 = property class="Bool (strict)"(reference=w266) -> ("Label.Text"=w265:string)  [unwired: 1 in, 2 out]
        n218 = local read "FPenAcon"() -> (w255:refnum<vi>[])
        n219 = call "SubVI Set Front panel elements.vi"("Enable elements (T)"=FALSE, "Array"=w255) -> ("error out"=w253:errorcluster)  [unwired: 9 in]
        n220 = Scan From String(format string="S%dC%d", input string=w265, error in=w253, default 1=w252, default 2=w252) -> (error out=w259:errorcluster, output 1=w263:i32, output 2=w262:i32)  [unwired: 1 in, 2 out]
        n221 = local read "VISA"() -> (w261:refnum<visa-resource-name>)
        n222 = call "Set Channel.vi"("Channel"=w262, "Channel Status"=w260, "Slave"=w263, "error in (no error)"=w259, "VISA resource name"=w261) -> ("error out"=w257:errorcluster, "VISA resource name out"=w251:refnum<visa-resource-name>)  [unwired: 5 in]
        n223 = local write "VISA"(w251) -> ()
        n224 = local read "FPenAcon"() -> (w258:refnum<vi>[])
        n225 = call "SubVI Set Front panel elements.vi"("error in (passthrough)"=w257, "Array"=w258) -> ("error out"=w256:errorcluster)  [unwired: 9 in]
        n226 = local write "error"(w256) -> ()
      }
      event "G1C1", "G1C2", "G2C1", "G2C2", "G3C1", "G3C2", "G4C1", "G4C2", "G5C1", "G5C2", "G6C1", "G6C2": Value Change {
        w274 = 0 ("default value 1")
        n227 = event-data() -> ("CtlRef"=w280:refnum<vi>, "NewVal"=w276:bool)  [unwired: 1 in, 4 out]
        n228 = property class="Bool (strict)"(reference=w280) -> ("Label.Text"=w282:string)  [unwired: 1 in, 2 out]
        n229 = local read "FPenAcon"() -> (w273:refnum<vi>[])
        n230 = call "SubVI Set Front panel elements.vi"("Enable elements (T)"=FALSE, "Array"=w273) -> ("error out"=w271:errorcluster)  [unwired: 9 in]
        n231 = Scan From String(format string="G%dC%d", input string=w282, error in=w271, default 1=w274, default 2=w274) -> (error out=w275:errorcluster, output 1=w278:i32, output 2=w279:i32)  [unwired: 1 in, 2 out]
        n232 = local read "VISA"() -> (w277:refnum<visa-resource-name>)
        n233 = call "Set Guard.vi"("Channel"=w279, "Channel Guard Status"=w276, "Slave"=w278, "error in (no error)"=w275, "VISA resource name"=w277) -> ("error out"=w269:errorcluster, "VISA resource name out"=w267:refnum<visa-resource-name>)  [unwired: 5 in]
        n234 = local write "VISA"(w267) -> ()
        n235 = local read "FPenAcon"() -> (w270:refnum<vi>[])
        n236 = call "SubVI Set Front panel elements.vi"("error in (passthrough)"=w269, "Array"=w270) -> ("error out"=w268:errorcluster)  [unwired: 9 in]
        n237 = local write "error"(w268) -> ()
      }
      event "Trigger source": Value Change {
        n238 = event-data() -> ()  [unwired: 1 in, 6 out]
        n239 = local read "FPenAcon"() -> (w291:refnum<vi>[])
        n240 = Equal?(x="Trigger source", y=enum32{"Internal", "External"}."External") -> (x = y?=w285:bool)
        n241 = call "SubVI Set Front panel elements.vi"("Enable elements (T)"=FALSE, "Array"=w291) -> ("error out"=w287:errorcluster)  [unwired: 9 in]
        n242 = local read "VISA"() -> (w289:refnum<visa-resource-name>)
        n243 = call "Configure Trigger Source.vi"("Trigger External (T)"=w285, "error in (no error)"=w287, "VISA resource name"=w289) -> ("error out"=w288:errorcluster, "VISA resource name out"=w283:refnum<visa-resource-name>)  [unwired: 7 in]
        n244 = local write "VISA"(w283) -> ()
        n245 = local read "FPenAcon"() -> (w292:refnum<vi>[])
        n246 = call "SubVI Set Front panel elements.vi"("error in (passthrough)"=w288, "Array"=w292) -> ("error out"=w293:errorcluster)  [unwired: 9 in]
        n247 = local write "error"(w293) -> ()
      }
      event "Trigger polarity": Value Change {
        n248 = event-data() -> ()  [unwired: 1 in, 6 out]
        n249 = local read "FPenAcon"() -> (w302:refnum<vi>[])
        n250 = Equal?(x="Trigger polarity", y=enum32{"Positive", "Negative"}."Positive") -> (x = y?=w296:bool)
        n251 = call "SubVI Set Front panel elements.vi"("Enable elements (T)"=FALSE, "Array"=w302) -> ("error out"=w300:errorcluster)  [unwired: 9 in]
        n252 = local read "VISA"() -> (w295:refnum<visa-resource-name>)
        n253 = call "Configure Trigger Polarity.vi"("Trigger Polarity Positive (T)"=w296, "error in (no error)"=w300, "VISA resource name"=w295) -> ("error out"=w299:errorcluster, "VISA resource name out"=w294:refnum<visa-resource-name>)  [unwired: 7 in]
        n254 = local write "VISA"(w294) -> ()
        n255 = local read "FPenAcon"() -> (w303:refnum<vi>[])
        n256 = call "SubVI Set Front panel elements.vi"("error in (passthrough)"=w299, "Array"=w303) -> ("error out"=w304:errorcluster)  [unwired: 9 in]
        n257 = local write "error"(w304) -> ()
      }
      event "timer set": Value Change {
        n258 = event-data() -> ()  [unwired: 1 in, 6 out]
        n259 = To Double Precision Float(number="Timer (ms)") -> (double precision float=w310:dbl)
        n260 = local read "FPenAcon"() -> (w313:refnum<vi>[])
        n261 = expression code="x/1000"(w310) -> (w309:dbl)
        n262 = call "SubVI Set Front panel elements.vi"("Enable elements (T)"=FALSE, "Array"=w313) -> ("error out"=w307:errorcluster)  [unwired: 9 in]
        n263 = local read "VISA"() -> (w308:refnum<visa-resource-name>)
        n264 = call "Configure Timer.vi"("error in (no error)"=w307, "Internal timer (2 s)"=w309, "VISA resource name"=w308) -> ("error out"=w306:errorcluster, "VISA resource name out"=w305:refnum<visa-resource-name>)  [unwired: 7 in]
        n265 = local write "VISA"(w305) -> ()
        n266 = local read "FPenAcon"() -> (w314:refnum<vi>[])
        n267 = call "SubVI Set Front panel elements.vi"("error in (passthrough)"=w306, "Array"=w314) -> ("error out"=w315:errorcluster)  [unwired: 9 in]
        n268 = local write "error"(w315) -> ()
      }
      event "timer get": Value Change {
        n269 = event-data() -> ()  [unwired: 1 in, 6 out]
        n270 = local read "FPenAcon"() -> (w323:refnum<vi>[])
        n271 = call "SubVI Set Front panel elements.vi"("Enable elements (T)"=FALSE, "Array"=w323) -> ("error out"=w321:errorcluster)  [unwired: 9 in]
        n272 = local read "VISA"() -> (w319:refnum<visa-resource-name>)
        n273 = call "Get Timer.vi"("error in (no error)"=w321, "VISA resource name"=w319) -> ("error out"=w320:errorcluster, "Internal Timer value (s)"=w318:dbl, "VISA resource name out"=w316:refnum<visa-resource-name>)  [unwired: 7 in]
        n274 = local write "VISA"(w316) -> ()
        n275 = local read "FPenAcon"() -> (w324:refnum<vi>[])
        n276 = expression code="int(x*1000)"(w318) -> (w317:dbl)
        n277 = call "SubVI Set Front panel elements.vi"("error in (passthrough)"=w320, "Array"=w324) -> ("error out"=w325:errorcluster)  [unwired: 9 in]
        n278 = local write "Timer (ms)"(w317) -> ()
        n279 = local write "error"(w325) -> ()
      }
      event "delay set": Value Change {
        n280 = event-data() -> ()  [unwired: 1 in, 6 out]
        n281 = local read "FPenAcon"() -> (w333:refnum<vi>[])
        n282 = expression code="x/1000"("Enable\nDelay (ms)") -> (w328:dbl)
        n283 = call "SubVI Set Front panel elements.vi"("Enable elements (T)"=FALSE, "Array"=w333) -> ("error out"=w330:errorcluster)  [unwired: 9 in]
        n284 = local read "VISA"() -> (w331:refnum<visa-resource-name>)
        n285 = call "Configure Delay.vi"("error in (no error)"=w330, "Delay (s)"=w328, "VISA resource name"=w331) -> ("error out"=w329:errorcluster, "VISA resource name out"=w326:refnum<visa-resource-name>)  [unwired: 7 in]
        n286 = local write "VISA"(w326) -> ()
        n287 = local read "FPenAcon"() -> (w334:refnum<vi>[])
        n288 = call "SubVI Set Front panel elements.vi"("error in (passthrough)"=w329, "Array"=w334) -> ("error out"=w335:errorcluster)  [unwired: 9 in]
        n289 = local write "error"(w335) -> ()
      }
      event "delay get": Value Change {
        n290 = event-data() -> ()  [unwired: 1 in, 6 out]
        n291 = local read "FPenAcon"() -> (w343:refnum<vi>[])
        n292 = call "SubVI Set Front panel elements.vi"("Enable elements (T)"=FALSE, "Array"=w343) -> ("error out"=w341:errorcluster)  [unwired: 9 in]
        n293 = local read "VISA"() -> (w339:refnum<visa-resource-name>)
        n294 = call "Get Delay.vi"("error in (no error)"=w341, "VISA resource name"=w339) -> ("error out"=w340:errorcluster, "Delay (s)"=w338:dbl, "VISA resource name out"=w336:refnum<visa-resource-name>)  [unwired: 7 in]
        n295 = local write "VISA"(w336) -> ()
        n296 = local read "FPenAcon"() -> (w344:refnum<vi>[])
        n297 = expression code="int(x*1000)"(w338) -> (w337:dbl)
        n298 = call "SubVI Set Front panel elements.vi"("error in (passthrough)"=w340, "Array"=w344) -> ("error out"=w345:errorcluster)  [unwired: 9 in]
        n299 = local write "Enable\nDelay (ms)"(w337) -> ()
        n300 = local write "error"(w345) -> ()
      }
      event "check channels", "dummy for event \"check channels\"": Value Change {
        # "this is only to get possibility\nto start this event case\neven if button \"check channels\"\nis latching"
        n301 = event-data() -> ()  [unwired: 1 in, 6 out]
        n302 = local read "FPenAcon"() -> (w362:refnum<vi>[])
        n303 = call "SubVI Set Front panel elements.vi"("Enable elements (T)"=FALSE, "Array"=w362) -> ("error out"=w355:errorcluster)  [unwired: 9 in]
        n304 = local read "VISA"() -> (w356:refnum<visa-resource-name>)
        n305 = local read "Guards ref array"() -> (w352:refnum<vi>[][])
        n306 = local read "Slaves ref array"() -> (w358:refnum<vi>[][])
        n307 = call "Get Slaves Number & Positions.vi"("error in (no error)"=w355, "VISA resource name"=w356) -> ("error out"=w353:errorcluster, "Connected Slaves"=w357:bool[], "No. of Slaves"=w359:u32, "VISA resource name out"=w347:refnum<visa-resource-name>)  [unwired: 6 in]
        "Connected\nboards" <- w357
        n308 = local write "No. of connected slave boards:"(w359) -> ()
        n309 = for {
          tunnel: w358 -> [w370] mode=indexing
          tunnel: w357 -> [w366] mode=indexing
          shift-right: [w367] -> w354
          shift-left: w353 -> [w369]
          tunnel: w352 -> [w365] mode=indexing
          n310 = call "SubVI Set Front panel elements.vi"("Enable elements (T)"=w366, "error in (passthrough)"=w369, "Array"=w370) -> ("error out"=w368:errorcluster)  [unwired: 8 in]
          n311 = call "SubVI Set Front panel elements.vi"("Enable elements (T)"=w366, "error in (passthrough)"=w368, "Array"=w365) -> ("error out"=w367:errorcluster)  [unwired: 8 in]
        }
        n312 = for {
          N: 2 -> [_]
          shift-right: [w376] -> w349
          shift-left: w354 -> [w375]
          shift-right: [w371] -> w346
          shift-left: w347 -> [w372]
          i -> [w374]
          n313 = Increment(x=w374) -> (x+1=w373:i32)
          n314 = for {
            N: 6 -> [_]
            shift-right: [w386] -> w376
            shift-left: w375 -> [w385]
            tunnel: w373 -> [w381]
            shift-right: [w378] -> w371
            shift-left: w372 -> [w379]
            i -> [w384]
            # "#XXX no way how to check guard status?"
            n315 = Increment(x=w384) -> (x+1=w382:i32)
            n316 = call "Get Channel Status.vi"("Channel"=w381, "Slave"=w382, "error in (no error)"=w385, "VISA resource name"=w379) -> ("error out"=w386:errorcluster, "Channel Enabled"=w380:bool, "VISA resource name out"=w378:refnum<visa-resource-name>)  [unwired: 5 in]
            n317 = local read "Slaves ref array"() -> (w383:refnum<vi>[][])
            n318 = call "SubVI Set FP Channel-Guard value.vi"("Value"=w380, "Ch ID"=w381, "Slave ID"=w382, "Slaves ref array"=w383) -> ()  [unwired: 7 in, 1 out]
          }
        }
        n319 = local write "VISA"(w346) -> ()
        n320 = Enqueue Element(queue=w350, element="slaves update", error in (no error)=w349) -> (error out=w348:errorcluster)  [unwired: 1 in, 2 out]
        n321 = local read "FPenAcon"() -> (w363:refnum<vi>[])
        n322 = call "SubVI Set Front panel elements.vi"("error in (passthrough)"=w348, "Array"=w363) -> ("error out"=w364:errorcluster)  [unwired: 9 in]
        n323 = local write "error"(w364) -> ()
      }
      event "Get Status": Value Change {
        n324 = event-data() -> ()  [unwired: 1 in, 6 out]
        n325 = local read "FPenAcon"() -> (w406:refnum<vi>[])
        n326 = call "SubVI Set Front panel elements.vi"("Enable elements (T)"=FALSE, "Array"=w406) -> ("error out"=w401:errorcluster)  [unwired: 9 in]
        n327 = local read "VISA"() -> (w402:refnum<visa-resource-name>)
        n328 = call "Get MX Status.vi"("error in (no error)"=w401, "VISA resource name"=w402) -> ("error out"=w400:errorcluster, "Ready?"=→"Ready?":bool, "Enabled"=→"Enabled":bool, "VISA resource name out"=w387:refnum<visa-resource-name>, "TRG Polarity Positive"=w395:bool, "Local?"=w399:bool, "TRG External"=w391:bool)  [unwired: 3 in]
        n329 = local write "VISA"(w387) -> ()
        n330 = local read "FPenAcon"() -> (w407:refnum<vi>[])
        n331 = Select(t=enum32{"Remote", "Local"}."Local" ("Operation"), s=w399, f=enum32{"Remote", "Local"}."Remote" ("Operation")) -> (s? t:f=w396:enum32{"Remote", "Local"})
        n332 = Select(t=enum32{"Positive", "Negative"}."Positive" ("Trigger polarity"), s=w395, f=enum32{"Positive", "Negative"}."Negative" ("Trigger polarity")) -> (s? t:f=w392:enum32{"Positive", "Negative"})
        n333 = Select(t=enum32{"Internal", "External"}."External" ("Trigger source"), s=w391, f=enum32{"Internal", "External"}."Internal" ("Trigger source")) -> (s? t:f=w388:enum32{"Internal", "External"})
        n334 = call "SubVI Set Front panel elements.vi"("error in (passthrough)"=w400, "Array"=w407) -> ("error out"=w408:errorcluster)  [unwired: 9 in]
        n335 = local write "Operation"(w396) -> ()
        n336 = local write "Trigger polarity"(w392) -> ()
        n337 = local write "Trigger source"(w388) -> ()
        n338 = local write "error"(w408) -> ()
      }
      event "no sequences get": Value Change {
        n339 = event-data() -> ()  [unwired: 1 in, 6 out]
        n340 = local read "FPenAcon"() -> (w415:refnum<vi>[])
        n341 = call "SubVI Set Front panel elements.vi"("Enable elements (T)"=FALSE, "Array"=w415) -> ("error out"=w413:errorcluster)  [unwired: 9 in]
        n342 = local read "VISA"() -> (w411:refnum<visa-resource-name>)
        n343 = call "Get Number of Sequences.vi"("error in (no error)"=w413, "VISA resource name"=w411) -> ("error out"=w412:errorcluster, "Number of sequences"=w410:i32, "VISA resource name out"=w409:refnum<visa-resource-name>)  [unwired: 7 in]
        n344 = local write "VISA"(w409) -> ()
        n345 = local read "FPenAcon"() -> (w416:refnum<vi>[])
        n346 = local write "Number of sequence lines:"(w410) -> ()
        n347 = call "SubVI Set Front panel elements.vi"("error in (passthrough)"=w412, "Array"=w416) -> ("error out"=w417:errorcluster)  [unwired: 9 in]
        n348 = local write "error"(w417) -> ()
      }
      event "sequence editor": Value Change {
        n349 = event-data() -> ()  [unwired: 1 in, 6 out]
        n350 = Enqueue Element(queue=w419, element="FP open") -> ()  [unwired: 2 in, 3 out]
      }
      event "Load sq to MX": Value Change {
        n351 = event-data() -> ()  [unwired: 1 in, 6 out]
        n352 = disable-structure shown="Default" {
          disable-tunnel: w424 -> [w457]
          disable-tunnel: [w442] -> w423
          disable-tunnel: [w441] -> w422
          frame Enabled {
            # "Get actual values from Sequence editor.vi"
            n353 = property class="VI"(reference=w457) -> ("Panel"=w456:refnum<vi>)  [unwired: 1 in, 2 out]
            n354 = property class="Pnl"(reference=w456) -> (reference out=w443:refnum<vi>, "Controls[]"=w444:refnum<vi>[])  [unwired: 1 in, 1 out]
            n355 = Close Reference(reference=w443) -> ()  [unwired: 1 in, 1 out]
            n356 = Close Reference(reference=w444) -> ()  [unwired: 1 in, 1 out]
            n357 = for {
              tunnel: w444 -> [w459] mode=indexing
              tunnel: [w458] -> w446 mode=indexing
              n358 = property class="Ctl"(reference=w459) -> ("Label.Text"=w458:string)  [unwired: 1 in, 2 out]
            }
            n359 = call "Search Unsorted 1D Array.vim"("element"="Sequence" ("Label.Text"), "unsorted 1D array"=w446) -> ("index of element"=w448:i32)  [unwired: 9 in]
            n360 = call "Search Unsorted 1D Array.vim"("element"="Timing\ndelay" ("Label.Text"), "unsorted 1D array"=w446) -> ("index of element"=w454:i32)  [unwired: 9 in]
            n361 = Index Array(array=w444, index=w448) -> (element=w449:refnum<vi>)
            n362 = property class="Ctl"(reference=w449) -> ("Value"=w450:variant)  [unwired: 1 in, 2 out]
            n363 = Index Array(array=w444, index=w454) -> (element=w453:refnum<vi>)
            n364 = property class="Ctl"(reference=w453) -> ("Value"=w452:variant)  [unwired: 1 in, 2 out]
            n365 = Variant To Data(type=u8[] [] ("Ch. bytes 2"), Variant=w452) -> (data=w441:u8[])  [unwired: 1 in, 1 out]
            n366 = Variant To Data(type=bool[][] [], Variant=w450) -> (data=w442:bool[][])  [unwired: 1 in, 1 out]
          }
        }
        n367 = Array Size(array=w422) -> (size(s)=w421:i32)
        n368 = Equal To 0?(x=w421) -> (x = 0?=w420:bool)
        n369 = case shown="False" w420 {
          tunnel: w423 -> [w431 _]
          tunnel: w422 -> [w430 _]
          frame False {
            n370 = local read "FPenAcon"() -> (w435:refnum<vi>[])
            n371 = call "Sequences to Bytes.vi"("Channel states"=w431) -> ("Ch. bytes 2"=w438:u8[], "Ch. bytes 1"=w439:u8[])  [unwired: 9 in]
            n372 = call "SubVI Set Front panel elements.vi"("Enable elements (T)"=FALSE, "Array"=w435) -> ("error out"=w433:errorcluster)  [unwired: 9 in]
            n373 = local read "VISA"() -> (w432:refnum<visa-resource-name>)
            n374 = call "Load Sequences.vi"("Byte 2 Ch."=w438, "Byte 3 Timing Delay"=w430, "Byte 1 Ch."=w439, "error in (no error)"=w433, "VISA resource name"=w432) -> ("error out"=w428:errorcluster, "VISA resource name out"=w426:refnum<visa-resource-name>)  [unwired: 5 in]
            n375 = local read "FPenAcon"() -> (w436:refnum<vi>[])
            n376 = call "Get Number of Sequences.vi"("error in (no error)"=w428, "VISA resource name"=w426) -> ("error out"=w427:errorcluster, "Number of sequences"=w429:i32, "VISA resource name out"=w425:refnum<visa-resource-name>)  [unwired: 7 in]
            n377 = call "SubVI Set Front panel elements.vi"("error in (passthrough)"=w427, "Array"=w436) -> ("error out"=w437:errorcluster)  [unwired: 9 in]
            n378 = local write "VISA"(w425) -> ()
            n379 = local write "error"(w437) -> ()
            n380 = local write "Number of sequence lines:"(w429) -> ()
          }
          frame True {
            n381 = One Button Dialog(message="Sequence matrix is empty.\nUse sequence editor to create\nsequence or load sequence\nfrom file.") -> ()  [unwired: 1 in, 1 out]
          }
        }
      }
      event "set sq line": Value Change {
        n382 = event-data() -> ()  [unwired: 1 in, 6 out]
        n383 = disable-structure shown="Default" {
          disable-tunnel: w474 -> [w485]
          disable-tunnel: [w475] -> w469
          frame Enabled {
            # "Get actual values from Sequence editor.vi"
            n384 = property class="VI"(reference=w485) -> ("Panel"=w484:refnum<vi>)  [unwired: 1 in, 2 out]
            n385 = property class="Pnl"(reference=w484) -> (reference out=w476:refnum<vi>, "Controls[]"=w477:refnum<vi>[])  [unwired: 1 in, 1 out]
            n386 = Close Reference(reference=w476) -> ()  [unwired: 1 in, 1 out]
            n387 = Close Reference(reference=w477) -> ()  [unwired: 1 in, 1 out]
            n388 = for {
              tunnel: w477 -> [w487] mode=indexing
              tunnel: [w486] -> w479 mode=indexing
              n389 = property class="Ctl"(reference=w487) -> ("Label.Text"=w486:string)  [unwired: 1 in, 2 out]
            }
            n390 = call "Search Unsorted 1D Array.vim"("element"="Sequence" ("Label.Text"), "unsorted 1D array"=w479) -> ("index of element"=w481:i32)  [unwired: 9 in]
            n391 = Index Array(array=w477, index=w481) -> (element=w482:refnum<vi>)
            n392 = property class="Ctl"(reference=w482) -> ("Value"=w483:variant)  [unwired: 1 in, 2 out]
            n393 = Variant To Data(type=bool[][] [], Variant=w483) -> (data=w475:bool[][])  [unwired: 1 in, 1 out]
          }
        }
        n394 = local read "FPenAcon"() -> (w472:refnum<vi>[])
        n395 = Decrement(x="Set to sequence line:") -> (x-1=w461:i32)
        n396 = Index Array(array=w469, index (row)=w461) -> (element=w468:bool[])  [unwired: 1 in]
        n397 = call "SubVI Set Front panel elements.vi"("Enable elements (T)"=FALSE, "Array"=w472) -> ("error out"=w470:errorcluster)  [unwired: 9 in]
        n398 = local read "VISA"() -> (w467:refnum<visa-resource-name>)
        n399 = call "Set Sequence Line.vi"("error in (no error)"=w470, "Sequence Line"=w468, "VISA resource name"=w467) -> ("error out"=w466:errorcluster, "VISA resource name out"=w460:refnum<visa-resource-name>)  [unwired: 7 in]
        n400 = local write "VISA"(w460) -> ()
        n401 = local read "FPenAcon"() -> (w473:refnum<vi>[])
        n402 = call "SubVI Set Front panel elements.vi"("error in (passthrough)"=w466, "Array"=w473) -> ("error out"=w465:errorcluster)  [unwired: 9 in]
        n403 = property on="dummy for event \"check channels\"" class="Bool (strict)"(error in=w465, "Val(Sgnl)"=TRUE) -> (error out=w464:errorcluster)  [unwired: 1 in, 1 out]
        n404 = local write "error"(w464) -> ()
      }
      event "Get sq from MX": Value Change {
        n405 = event-data() -> ()  [unwired: 1 in, 6 out]
        n406 = local read "FPenAcon"() -> (w490:refnum<vi>[])
        n407 = call "SubVI Set Front panel elements.vi"("Enable elements (T)"=FALSE, "Array"=w490) -> ("error out"=w508:errorcluster)  [unwired: 9 in]
        n408 = local read "VISA"() -> (w506:refnum<visa-resource-name>)
        n409 = call "Get Sequences.vi"("error in (no error)"=w508, "VISA resource name"=w506) -> ("error out"=w507:errorcluster, "VISA resource name out"=w488:refnum<visa-resource-name>, "Byte 3 Delay"=w500:u8[], "Byte 2 Ch."=w503:u8[], "Byte 1 Ch."=w504:u8[])  [unwired: 5 in]
        n410 = local write "VISA"(w488) -> ()
        n411 = Array Size(array=w500) -> (size(s)=w505:i32)
        n412 = local read "FPenAcon"() -> (w509:refnum<vi>[])
        n413 = call "Bytes to Sequences.vi"("Ch. bytes 2"=w503, "Ch. bytes 1"=w504) -> ("Array"=w501:bool[][])  [unwired: 9 in]
        n414 = call "SubVI Set Front panel elements.vi"("error in (passthrough)"=w507, "Array"=w509) -> ("error out"=w510:errorcluster)  [unwired: 9 in]
        n415 = local write "Number of sequence lines:"(w505) -> ()
        n416 = local write "error"(w510) -> ()
        n417 = disable-structure shown="Default" {
          disable-tunnel: w502 -> [w524]
          disable-tunnel: w501 -> [w513]
          disable-tunnel: w500 -> [w512]
          disable-tunnel: w499 -> [w511]
          disable-tunnel: [w511] -> w491
          frame Enabled {
            # "Push actual values to Sequence editor.vi"
            n418 = property class="VI"(reference=w524) -> ("Panel"=w523:refnum<vi>)  [unwired: 1 in, 2 out]
            n419 = property class="Pnl"(reference=w523) -> (reference out=w514:refnum<vi>, "Controls[]"=w515:refnum<vi>[])  [unwired: 1 in, 1 out]
            n420 = Close Reference(reference=w514) -> ()  [unwired: 1 in, 1 out]
            n421 = Close Reference(reference=w515) -> ()  [unwired: 1 in, 1 out]
            n422 = for {
              tunnel: w515 -> [w526] mode=indexing
              tunnel: [w525] -> w516 mode=indexing
              n423 = property class="Ctl"(reference=w526) -> ("Label.Text"=w525:string)  [unwired: 1 in, 2 out]
            }
            n424 = call "Search Unsorted 1D Array.vim"("element"="Sequence" ("Label.Text"), "unsorted 1D array"=w516) -> ("index of element"=w518:i32)  [unwired: 9 in]
            n425 = call "Search Unsorted 1D Array.vim"("element"="Timing\ndelay" ("Label.Text"), "unsorted 1D array"=w516) -> ("index of element"=w521:i32)  [unwired: 9 in]
            n426 = Index Array(array=w515, index=w518) -> (element=w519:refnum<vi>)
            n427 = property class="Ctl"(reference=w519, "Value"=w513) -> ()  [unwired: 1 in, 2 out]
            n428 = Index Array(array=w515, index=w521) -> (element=w520:refnum<vi>)
            n429 = property class="Ctl"(reference=w520, "Value"=w512) -> ()  [unwired: 1 in, 2 out]
          }
        }
        n430 = Enqueue Element(queue=w491, element="sequence fill missing collumns") -> (queue out=w495:refnum<queue>, error out=w498:errorcluster)  [unwired: 2 in, 1 out]
        n431 = Enqueue Element(queue=w495, element="index timing update", error in (no error)=w498) -> (queue out=w496:refnum<queue>, error out=w497:errorcluster)  [unwired: 1 in, 1 out]
        n432 = Enqueue Element(queue=w496, element="scrollbar sync", error in (no error)=w497) -> ()  [unwired: 1 in, 3 out]
      }
    }
  }
  n433 = flat-sequence {
    tunnel: w11 -> [w530]
    tunnel: w12 -> [w527]
    tunnel: w15 -> [_]
    tunnel: [w530] -> w4
    tunnel: [w528] -> w2
    tunnel: w4 -> [w534]
    tunnel: [w534] -> w3
    tunnel: w2 -> [w533]
    tunnel: [w532] -> w1
    tunnel: [w537] -> w8
    tunnel: w3 -> [w537]
    tunnel: [w536] -> w7
    tunnel: w1 -> [w536]
    tunnel: w8 -> [w541]
    tunnel: w7 -> [w539]
    frame #0 {
      # "send signal\nto quit\nMX sequence panel"
      n434 = Enqueue Element(queue=w527, element="quit") -> (error out=w528:errorcluster)  [unwired: 2 in, 2 out]
    }
    frame #1 {
      # "give panel \nchance to quit\nby itself"
      n435 = call "Stall Data Flow.vim"("value in"=w533, "milliseconds to wait"=u32 50) -> ("value out"=w532:errorcluster)  [unwired: 1 out]
    }
    frame #2 {
      # "ensure panel\nis closed"
      n436 = invoke class="VI" method="FP.Close"(reference=w537) -> (error out=w535:errorcluster)  [unwired: 2 in, 2 out]
      n437 = call <vilib>:"Clear Errors.vi"("error in (no error)"=w535) -> ()  [unwired: 5 in, 2 out]
    }
    frame #3 {
      # "quit this VI if runtime or just stop\nif developement"
      n438 = property on="connect" class="Bool"() -> ("DisabledEnum"=w538:T1)  [unwired: 2 in, 2 out]
      n439 = case shown="\"Disabled\"" w538 {
        tunnel: [errorcluster {"status"=FALSE, "code"=0, "source"=""} ("error out") w545] -> w543
        frame "Enabled", Default {
        }
        frame "Disabled" {
          # "disconnect\nonly if connection was\nnot innitiated"
          n440 = local read "VISA"() -> (w546:refnum<visa-resource-name>)
          n441 = call "Close.vi"("VISA resource name"=w546) -> ("error out"=w545:errorcluster)  [unwired: 10 in]
        }
      }
      n442 = Close Reference(reference=w541) -> (error out=w540:errorcluster)  [unwired: 1 in]
      n443 = Merge Errors(w543, w539, w540) -> (w542:errorcluster)
      "error" <- w542
      n444 = disable-structure shown="RUN_TIME_ENGINE==True" {
        disable-tunnel: w542 -> [_ _]
        frame condition #0 (active) {
          n445 = Stop(stop? (T)=TRUE) -> ()
        }
        frame condition #1 {
          n446 = Quit LabVIEW(quit? (T)=TRUE) -> ()
        }
      }
    }
  }
